vi "Joystick Drive.vi"   [LabVIEW 2013]
types:
  T1 = typedef "WPI_JoystickButtonState.ctl" = cluster{"Button 1":bool, "Button 2":bool, "Button 3":bool, "Button 4":bool, "Button 5":bool, "Button 6":bool, "Button 7":bool, "Button 8":bool, "Button 9":bool, "Button 10":bool, "Button 11":bool, "Button 12":bool}
  T2 = cluster{"Axes":cluster{"X Axis":dbl, "Y Axis":dbl, "Twist-Handle":dbl, "Throttle":dbl, "Unused":dbl, "Unused":dbl}, "Buttons":T1}
  T3 = cluster{"X Axis":dbl, "Y Axis":dbl, "Twist-Handle":dbl, "Throttle":dbl, "Unused":dbl, "Unused":dbl}
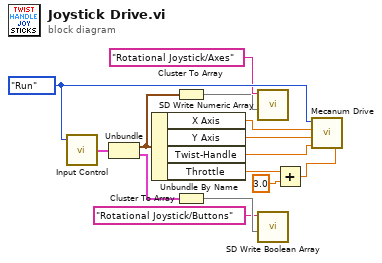
[diagram p0: block diagram]
diagram:
  w12 = enum16{"Open", "Run", "End"}."Run" ("State")
  n1 = call "Input Control.vi"("State"=w12) -> ("Twist-handle Joystick"=w14:T2)  [unwired: 2 in, 2 out]
  n2 = Unbundle(w14) -> ("Axes"=w5:T3, "Buttons"=w8:T1)
  n3 = Unbundle By Name(w5) -> ("X Axis"=w3:dbl, "Y Axis"=w4:dbl, "Twist-Handle"=w1:dbl, "Throttle"=w10:dbl)
  n4 = Cluster To Array(cluster=w5) -> (array=w6:dbl[])
  n5 = Cluster To Array(cluster=w8) -> (array=w9:bool[])
  n6 = call <vilib>:"SD Write Numeric Array.vi"("Numeric Array"=w6, "Name"="Rotational Joystick/Axes") -> ()  [unwired: 8 in, 2 out]
  n7 = call <vilib>:"SD Write Boolean Array.vi"("Boolean Array"=w9, "Name"="Rotational Joystick/Buttons") -> ()  [unwired: 8 in, 2 out]
  n8 = Add(x=w10, y=3.0) -> (x+y=w2:dbl)
  n9 = call "Mecanum Drive.vi"("Division"=w2, "Turning"=w1, "F/R"=w4, "Strafing"=w3, "State Control"=w12) -> ()  [unwired: 3 in]
